vi "transmit_can_pdo.vi"(11 "index":u16) -> (3 "return":i16)   [LabVIEW 2011]
uses:
  canopen_dll_master.dll
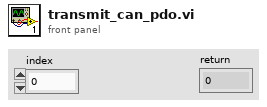
[diagram p1: front panel]
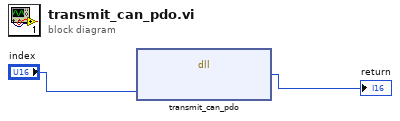
[diagram p0: block diagram]
diagram:
  n1 = dll-call lib="canopen_dll_master.dll" fn="transmit_can_pdo"("index"="index") -> ("return type"=→"return":i16)  [unwired: 4 in, 2 out]
